vi "test Script Analog Replay.vi"(8 "error in (no error)":errorcluster, 11 "TestCase in":refnum<class "Scripting API Test Case.lvclass">) -> (0 "error out":errorcluster, 3 "TestCase out":refnum<class "Scripting API Test Case.lvclass">)   [LabVIEW 2015, in "Scripting API Test Case.lvclass"]
uses:
  Scripting API Test Case.lvclass
  SysDef API/Engine Simulation Toolkit Custom Device Settings.ctl
  <vilib>/NI Veristand/Custom Device API/Custom Device Timed Loop Priority.ctl
  SysDef API/Analog Replay Settings.ctl
  SysDef API/Analog Replay Data Options.ctl
  System Explorer/FPGA Mem Size.ctl
  System Explorer/Position Reference.ctl
  System Explorer/Data Replay Data Selection Method.ctl
  NationalInstruments.VeriStand.SystemDefinitionAPI
  <userlib>/_OpenG.lib/file/file.llb/Append Path to Root if Relative - Scalar__ogtk.vi
  <vilib>/addons/_JKI Toolkits/VI Tester/TestCase.llb/TestCase.lvclass
  SysDef API/Engine Simulation Toolkit SysDef API.lvlib
  <vilib>/NI VeriStand/Custom Device API/Custom Device API.lvlib
  niveristand-custom-device-testing-tools/VeriStandTestUtilities/VeriStandTestUtilities.lvlib
  System Explorer/Engine Simulation Toolkit System Explorer.lvlib
panel:
  out "string":string
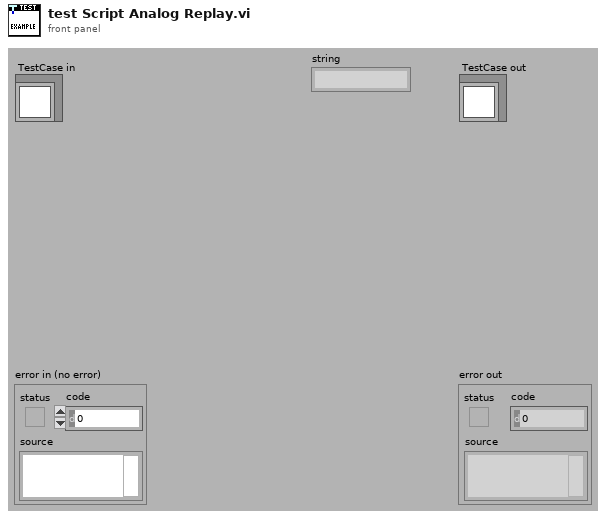
[diagram p1: front panel]
types:
  T1 = typedef "Engine Simulation Toolkit SysDef API.lvlib/Analog Replay Data Options.ctl" = cluster{"Input file":path, "Group":string, "Channel":string, "Reverse":bool, "FPGA Memory Size":T2, "Position reference":T3, "Data selection method":T4, "Offset":i32, "Samples":i32, "Missing teeth location":dbl, "DataPlugin":string}
  T2 = typedef "Engine Simulation Toolkit System Explorer.lvlib/FPGA Mem Size.ctl" = enum16{"65,536", "32,768", "16,384", "8,192", "4,096", "2,048", "1,024"}
  T3 = typedef "Engine Simulation Toolkit System Explorer.lvlib/Position Reference.ctl" = enum16{"Crank angle", "Cycle angle"}
  T4 = typedef "Engine Simulation Toolkit System Explorer.lvlib/Data Replay Data Selection Method.ctl" = enum32{"Manual", "AutoVRCrank"}
  T5 = typedef "Engine Simulation Toolkit SysDef API.lvlib/Analog Replay Settings.ctl" = cluster{"Name":string, "DAC bipolar range (V)":dbl, "Voltage below min speed":dbl, "Min speed (RPM)":dbl, "Voltage at min speed":dbl, "Max speed (RPM)":dbl, "Voltage at max speed":dbl, "Negate playback voltage values at negative engine speed":bool, "Allow run-time override of voltage scaling":bool}
  T6 = typedef "Engine Simulation Toolkit SysDef API.lvlib/Engine Simulation Toolkit Custom Device Settings.ctl" = cluster{"Name":string, "Execution priority":T7, "Rate decimation":i32, "CPU":i32, "Device address":string, "Bitfile path":path, "APUs":string[]}
  T7 = typedef "Custom Device API.lvlib/Custom Device Timed Loop Priority.ctl" = enum32{"Low", "Medium", "High"}
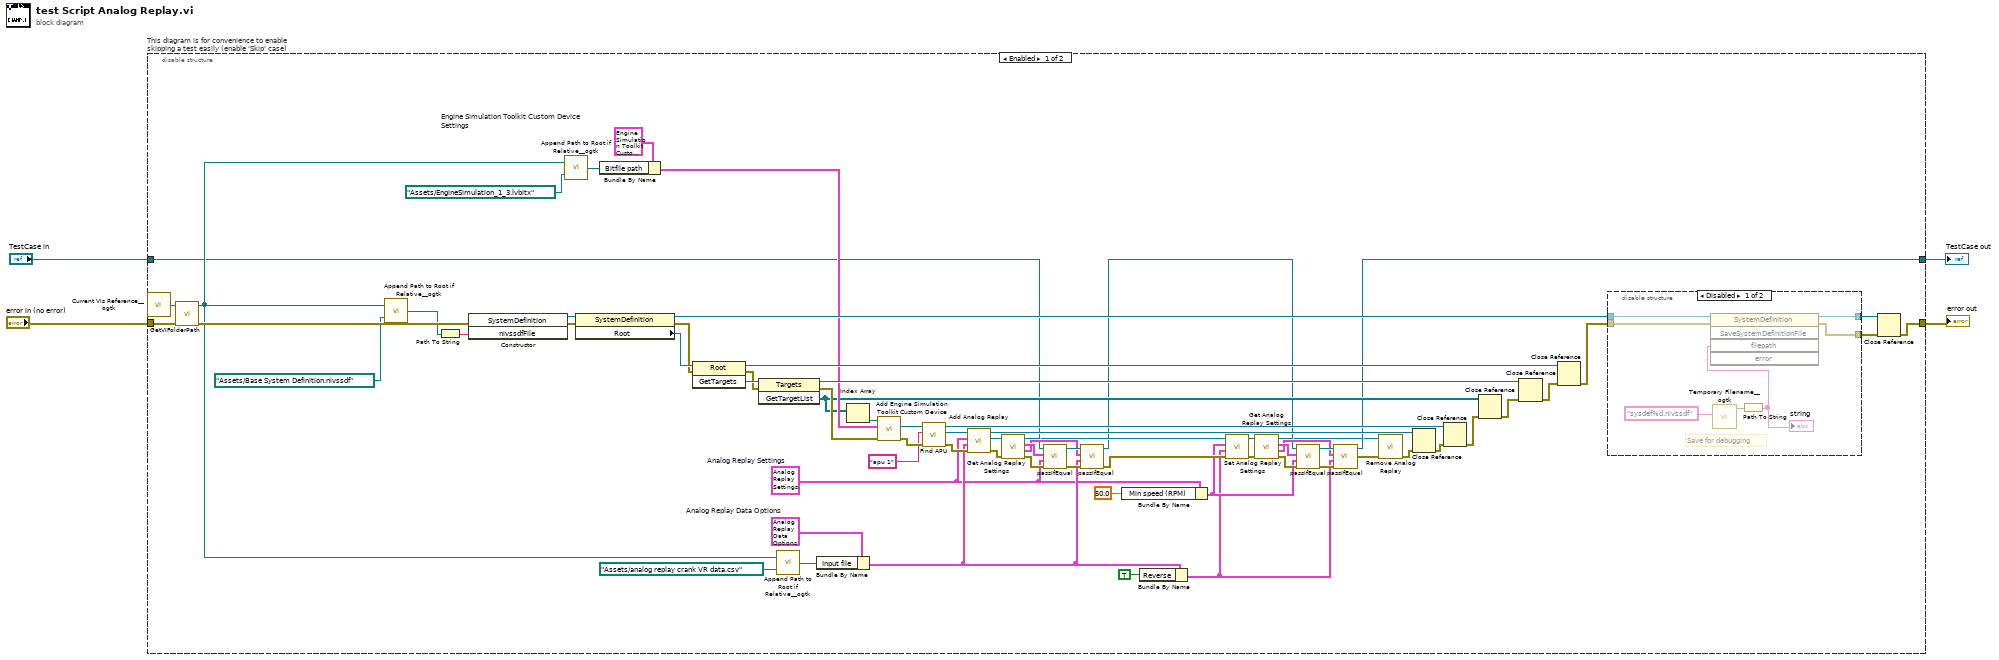
[diagram p0: block diagram]
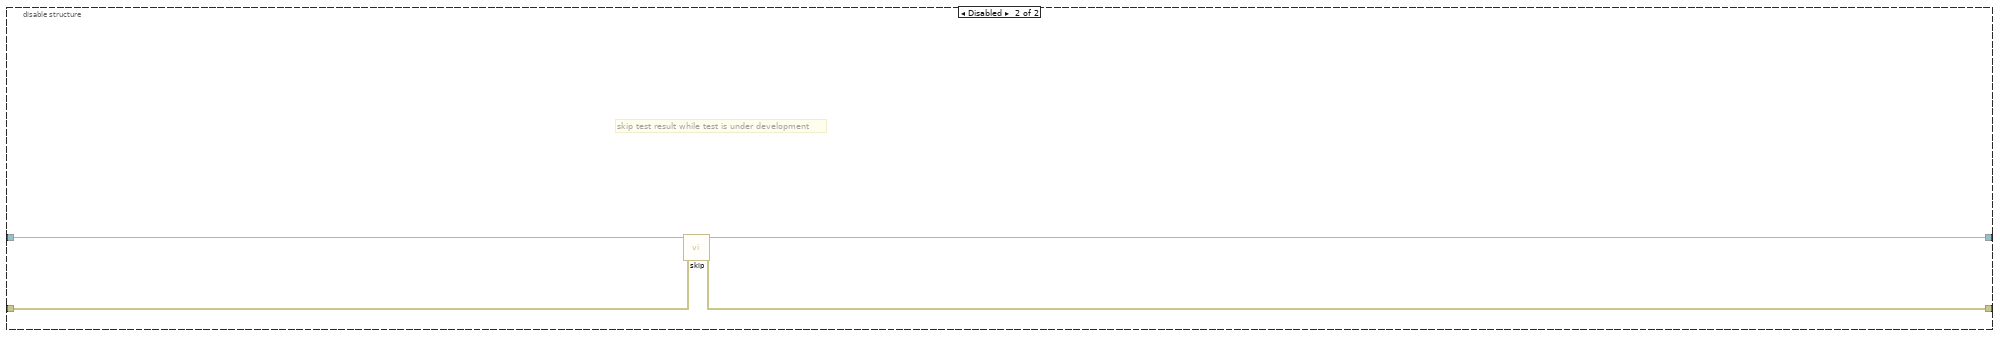
[diagram p3: hidden frame]
diagram:
  n1 = disable-structure "This diagram is for convenience to enable skipping a test easily (enable 'Skip' case)" shown="Enabled" {
    disable-tunnel: "TestCase in" -> [w25 w86]
    disable-tunnel: [w15 w84] -> w1
    disable-tunnel: [w65 w85] -> w3
    disable-tunnel: "error in (no error)" -> [w51 w83]
    frame Enabled {
      w40 = T1 {"Input file"=path "", "Group"="analog replay crank VR data", "Channel"="Ch0", "Reverse"=FALSE, "FPGA Memory Size"=enum."16,384", "Position reference"=enum."Crank angle", "Data selection method"=enum."Manual", "Offset"=50, "Samples"=100000, "Missing teeth location"=0.0, "DataPlugin"="CSV"}  # Analog Replay Data Options
      w11 = T5 {"Name"="replay AO 0", "DAC bipolar range (V)"=10.0, "Voltage below min speed"=0.5, "Min speed (RPM)"=1000.0, "Voltage at min speed"=1.0, "Max speed (RPM)"=10000.0, "Voltage at max speed"=10.0, "Negate playback voltage values at negative engine speed"=TRUE, "Allow run-time override of voltage scaling"=FALSE}  # Analog Replay Settings
      w67 = T6 {"Name"="Engine Simulation Toolkit", "Execution priority"=enum."Medium", "Rate decimation"=1, "CPU"=-2, "Device address"="RIO 0", "Bitfile path"=path "", "APUs"=[]}  # Engine Simulation Toolkit Custom Device Settings
      n2 = call <userlib>:"Current VIs Reference__ogtk.vi"() -> ("Current VI's reference"=w52:refnum<vi>)  [unwired: 5 in]
      n3 = call "GetVIFolderPath.vi"("error in (no error)"=w51, "VI Reference in"=w52) -> ("error out"=w50:errorcluster, "VI Folder Path out"=w37:path)  [unwired: 8 in]
      n4 = call-poly <userlib>:"Append Path to Root if Relative__ogtk.vi"("Absolute or Relative Path"=path "Assets/Base System Definition.nivssdf", "Root Path"=w37) -> ("Absolute or Appended Path"=w48:path)
      n5 = Path To String(path=w48) -> (string=w53:string)
      n6 = constructor class="SystemDefinition"(error in=w50, "nivssdfFile"=w53) -> (reference out=w73:refnum<k24>, error out=w72:errorcluster)  [unwired: 2 in, 2 out]
      n7 = call-poly <userlib>:"Append Path to Root if Relative__ogtk.vi"("Absolute or Relative Path"=path "Assets/EngineSimulation_1_3.lvbitx", "Root Path"=w37) -> ("Absolute or Appended Path"=w54:path)
      n8 = property class="SystemDefinition"(reference=w73, error in=w72) -> (reference out=w66:refnum<k24>, error out=w68:errorcluster, "Root"=w71:refnum<k24>)
      n9 = Bundle By Name(cluster=w67, "Bitfile path"=w54) -> (w56:T6)
      n10 = invoke class="Root" method="GetTargets"(reference=w71, error in=w68) -> (reference out=w61:refnum<k24>, error out=w69:errorcluster, "GetTargets"=w70:refnum<k24>)  [unwired: 1 in]
      n11 = invoke class="Targets" method="GetTargetList"(reference=w70, error in=w69) -> (reference out=w60:refnum<k24>, error out=w57:errorcluster, "GetTargetList"=w45:refnum<k24>[])  [unwired: 1 in]
      n12 = call-poly <userlib>:"Append Path to Root if Relative__ogtk.vi"("Absolute or Relative Path"=path "Assets/analog replay crank VR data.csv", "Root Path"=w37) -> ("Absolute or Appended Path"=w39:path)
      n13 = Bundle By Name(cluster=w40, "Input file"=w39) -> (w13:T1)
      n14 = Index Array(array=w45) -> (element=w47:refnum<k24>)  [unwired: 1 in]
      n15 = call "Add Engine Simulation Toolkit Custom Device.vi"("error in (no error)"=w57, "Engine Simulation Toolkit Custom Device Settings"=w56, "Target in"=w47) -> ("error out"=w43:errorcluster, "EST Custom Device"=w44:refnum<k24>)  [unwired: 6 in, 1 out]
      n16 = call "Find APU.vi"("error in (no error)"=w43, "APU name"="apu 1", "EST custom device in"=w44) -> ("error out"=w42:errorcluster, "APU Node"=w41:refnum<k24>, "EST custom device out"=w36:refnum<k24>)  [unwired: 6 in]
      n17 = call "Add Analog Replay.vi"("error in (no error)"=w42, "Analog Replay Data Options"=w13, "Analog Replay Settings"=w11, "APU Node in"=w41) -> ("error out"=w32:errorcluster, "Analog Replay out"=w33:refnum<k24>, "APU Node out"=w31:refnum<k24>)  [unwired: 5 in]
      n18 = call "Get Analog Replay Settings.vi"("error in (no error)"=w32, "Analog Replay in"=w33) -> ("error out"=w30:errorcluster, "Analog Replay Data Options"=w26:T1, "Analog Replay Settings"=w29:T5, "Analog Replay out"=w17:refnum<k24>)  [unwired: 6 in]
      n19 = call-dynamic "passIfEqual.vi"("error in (no error)"=w30, "y"=w11, "x"=w29, "TestCase in"=w25) -> ("error out"=w28:errorcluster, "TestCase out"=w27:refnum<class "Scripting API Test Case.lvclass">)  [unwired: 6 in]
      n20 = call-dynamic "passIfEqual.vi"("error in (no error)"=w28, "y"=w13, "x"=w26, "TestCase in"=w27) -> ("error out"=w16:errorcluster, "TestCase out"=w14:refnum<class "Scripting API Test Case.lvclass">)  [unwired: 6 in]
      n21 = Bundle By Name(cluster=w11, "Min speed (RPM)"=50.0) -> (w9:T5)
      n22 = Bundle By Name(cluster=w13, "Reverse"=TRUE) -> (w8:T1)
      n23 = call "Set Analog Replay Settings.vi"("error in (no error)"=w16, "Analog Replay Data Options"=w8, "Analog Replay Settings"=w9, "Analog Replay in"=w17) -> ("error out"=w19:errorcluster, "Analog Replay out"=w18:refnum<k24>)  [unwired: 6 in]
      n24 = call "Get Analog Replay Settings.vi"("error in (no error)"=w19, "Analog Replay in"=w18) -> ("error out"=w24:errorcluster, "Analog Replay Data Options"=w20:T1, "Analog Replay Settings"=w23:T5, "Analog Replay out"=w5:refnum<k24>)  [unwired: 6 in]
      n25 = call-dynamic "passIfEqual.vi"("error in (no error)"=w24, "y"=w9, "x"=w23, "TestCase in"=w14) -> ("error out"=w22:errorcluster, "TestCase out"=w21:refnum<class "Scripting API Test Case.lvclass">)  [unwired: 6 in]
      n26 = call-dynamic "passIfEqual.vi"("error in (no error)"=w22, "y"=w8, "x"=w20, "TestCase in"=w21) -> ("error out"=w7:errorcluster, "TestCase out"=w15:refnum<class "Scripting API Test Case.lvclass">)  [unwired: 6 in]
      n27 = call "Remove Analog Replay.vi"("error in (no error)"=w7, "Analog Replay in"=w5) -> ("error out"=w6:errorcluster)  [unwired: 9 in]
      n28 = Close Reference(reference=w31, error in (no error)=w6) -> (error out=w34:errorcluster)
      n29 = Close Reference(reference=w36, error in (no error)=w34) -> (error out=w46:errorcluster)
      n30 = Close Reference(reference=w45, error in (no error)=w46) -> (error out=w58:errorcluster)
      n31 = Close Reference(reference=w60, error in (no error)=w58) -> (error out=w59:errorcluster)
      n32 = Close Reference(reference=w61, error in (no error)=w59) -> (error out=w62:errorcluster)
      n33 = disable-structure shown="Disabled" {
        disable-tunnel: w66 -> [w80 w81]
        disable-tunnel: [w79 w82] -> w64
        disable-tunnel: [w78 w81] -> w63
        disable-tunnel: w62 -> [w77 w82]
        frame Disabled {
          # "Save for debugging"
          n34 = call <userlib>:"Temporary Filename__ogtk.vi"("pattern (lvtemp%d.tmp)"="sysdef%d.nivssdf") -> ("file in tmp dir"=w75:path)  [unwired: 5 in, 1 out]
          n35 = Path To String(path=w75) -> (string=w74:string)
          "string" <- w74
          n36 = invoke class="SystemDefinition" method="SaveSystemDefinitionFile"(reference=w80, error in=w77, "filepath"=w74) -> (reference out=w78:refnum<k24>, error out=w79:errorcluster)  [unwired: 2 in, 3 out]
        }
        frame Enabled {
        }
      }
      n37 = Close Reference(reference=w63, error in (no error)=w64) -> (error out=w65:errorcluster)
    }
    frame Disabled {
      # "skip test result while test is under development"
      n38 = call <vilib>:"skip.vi"("error in (no error)"=w83, "TestCase in"=w86) -> ("error out"=w85:errorcluster, "TestCase out"=w84:refnum<class "Scripting API Test Case.lvclass">)  [unwired: 8 in]
    }
  }
  "error out" <- w3
  "TestCase out" <- w1
